vi "CMDstr.vi"(9 "Test Type":enum16{"Voltage", "Current", "Power", "Frq"}(ring), 11 "Address":u8) -> (3 "CMD":string)   [LabVIEW 2015]
panel:
  out "CMD数组":u8[](array[numeric]) format="%.0x"
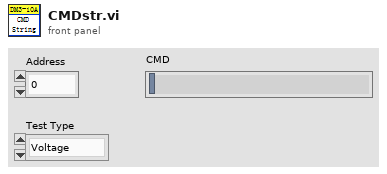
[diagram p1: front panel]
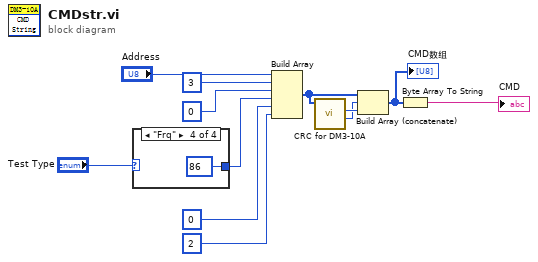
[diagram p0: block diagram]
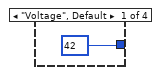
[diagram p2: hidden frame]
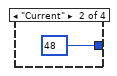
[diagram p3: hidden frame]
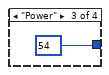
[diagram p4: hidden frame]
diagram:
  n1 = case shown="\"Frq\"" "Test Type" {
    tunnel: [u8 42 ("元素") u8 48 ("元素") u8 54 ("元素") u8 86 ("元素")] -> w9
    frame "Voltage", Default {
    }
    frame "Current" {
    }
    frame "Power" {
    }
    frame "Frq" {
    }
  }
  n2 = Build Array("Address", u8 3 ("元素"), u8 0 ("元素"), w9, u8 0 ("元素"), u8 2 ("元素")) -> (w6:u8[])
  n3 = call "CRC for DM3-10A.vi"("CMD"=w6) -> ("CRCLo"=w4:u8, "CRCHi"=w5:u8)  [unwired: 8 in, 1 out]
  n4 = Build Array (concatenate)(w6, w4, w5) -> (w3:u8[])
  "CMD数组" <- w3
  n5 = Byte Array To String(unsigned byte array=w3) -> (string=→"CMD":string)
